vi "PSVCH_Core Data.vi"(6 "Oper":enum16{"Init", "Read", "Write"}(ring)=enum."Read", 8 "Error In (no error)":errorcluster, 11 "VCH In":T1) -> (0 "Error Out":errorcluster, 3 "VCH Out":T1)   [LabVIEW 2016]
uses:
  Private/Ctrls/PSVCH_VCH Info.ctl
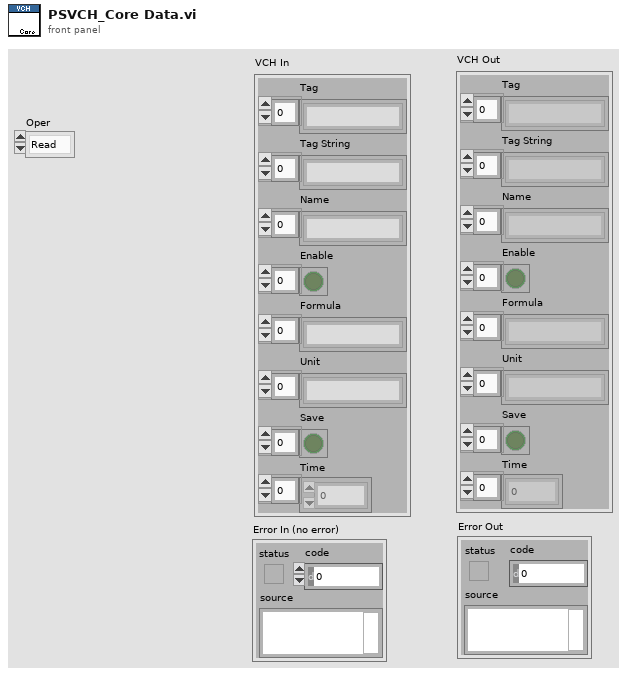
[diagram p1: front panel]
types:
  T1 = typedef "PSVCH_VCH Info.ctl" = cluster{"Tag":string[], "Tag String":string[], "Name":string[], "Enable":bool[], "Formula":string[], "Unit":string[], "Save":bool[], "Time":i64[]}
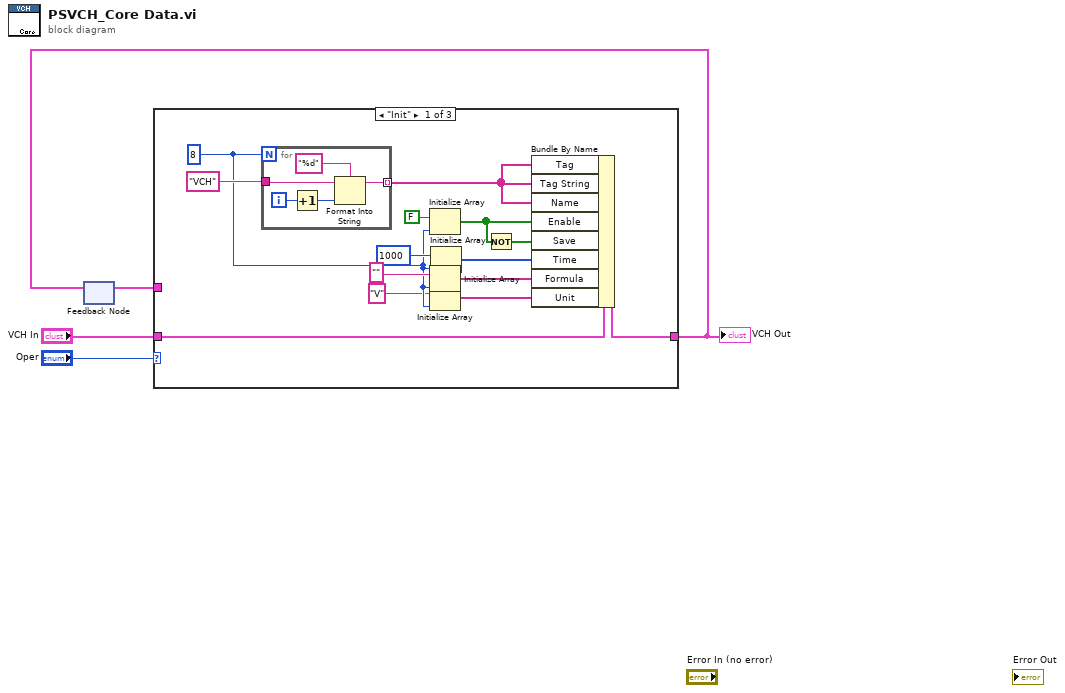
[diagram p0: block diagram]
diagram:
  n1 = feedback #1() -> (w3:T1)  [unwired: 1 in]
  n2 = case shown="\"Init\"" "Oper" {
    tunnel: "VCH In" -> [w9 _ w25]
    tunnel: [w8 w24 w25] -> w2
    tunnel: w3 -> [_ w24 _]
    frame "Init" {
      w7 = 8
      n3 = for {
        N: w7 -> [_]
        tunnel: "VCH" -> [w22]
        tunnel: [w19] -> w17 mode=indexing
        i -> [w23]
        n4 = Increment(x=w23) -> (x+1=w20:i32)
        n5 = Format Into String(format string="%d" ("格式字符串"), initial string=w22, w20) -> (resulting string=w19:string)  [unwired: 1 in, 1 out]
      }
      n6 = Initialize Array(FALSE ("布尔"), w7) -> (w11:bool[])
      n7 = Initialize Array("", w7) -> (w14:string[])
      n8 = Initialize Array("V", w7) -> (w5:string[])
      n9 = Initialize Array(i64 1000 ("Time"), w7) -> (w12:i64[])
      n10 = Not(x=w11) -> (.not. x?=w10:bool[])
      n11 = Bundle By Name(cluster=w9, "Tag"=w17, "Tag String"=w17, "Name"=w17, "Enable"=w11, "Save"=w10, "Time"=w12, "Formula"=w14, "Unit"=w5) -> (w8:T1)
    }
    frame "Read" {
    }
    frame "Write" {
    }
  }
  "VCH Out" <- w2
  n12 = feedback-in #1(w2) -> ()
